vi "TEST - Remove Duplicates from 1D Array.vi"(8 "error in (no error)":errorcluster) -> (0 "error out":errorcluster, 2 "Pass?":bool=TRUE)   [LabVIEW 2020]
doc: "This VI template can be used for the functional testing of VIs; this implementation includes handling for the testing of polymorphic VIs, and the polymorphic elements should be removed if not needed.\n\nCoded by Douglas A. Femec, January 24, 2006.\n\nCopyright (c) 2005-2006 MKS Instruments, Inc.\nAll rights reserved."
uses:
  TEST - Remove Duplicates from 1D Array - Inputs.ctl
  Polymorphizer+ Data Type.ctl
  TEST - Remove Duplicates from 1D Array - Outputs.ctl
  source/library/Remove Duplicates from 1D Array/Remove Duplicates from 1D Array (EXT).vi
  source/library/Remove Duplicates from 1D Array/Remove Duplicates from 1D Array (I64).vi
  source/library/Remove Duplicates from 1D Array/Remove Duplicates from 1D Array (U64).vi
  source/library/Remove Duplicates from 1D Array/Remove Duplicates from 1D Array (LVObject).vi
  source/library/Remove Duplicates from 1D Array/Remove Duplicates from 1D Array (DBL).vi
  source/library/Remove Duplicates from 1D Array/Remove Duplicates from 1D Array (SGL).vi
  source/library/Remove Duplicates from 1D Array/Remove Duplicates from 1D Array (I32).vi
  source/library/Remove Duplicates from 1D Array/Remove Duplicates from 1D Array (I16).vi
  source/library/Remove Duplicates from 1D Array/Remove Duplicates from 1D Array (I8).vi
  source/library/Remove Duplicates from 1D Array/Remove Duplicates from 1D Array (U32).vi
  source/library/Remove Duplicates from 1D Array/Remove Duplicates from 1D Array (U16).vi
  source/library/Remove Duplicates from 1D Array/Remove Duplicates from 1D Array (U8).vi
  source/library/Remove Duplicates from 1D Array/Remove Duplicates from 1D Array (CXT).vi
  source/library/Remove Duplicates from 1D Array/Remove Duplicates from 1D Array (CDB).vi
  source/library/Remove Duplicates from 1D Array/Remove Duplicates from 1D Array (CSG).vi
  source/library/Remove Duplicates from 1D Array/Remove Duplicates from 1D Array (String).vi
  source/library/Remove Duplicates from 1D Array/Remove Duplicates from 1D Array (Path).vi
  source/library/Remove Duplicates from 1D Array/Remove Duplicates from 1D Array (Variant).vi
  source/library/Remove Duplicates from 1D Array/Remove Duplicates from 1D Array (Boolean).vi
  TestClass/TestClass.lvclass
panel:
  out "Generated Outputs":T1[][](array[typedef]) {"Duplicate-Free Array Out" format="%.2f"}
  in  "Expected Outputs":T1[](array[typedef])=[{"Description"="Expect empty array", "Duplicate-Free Array Out"=[], "Indices of Removed Elements"=[]}, {"Description"="Array with one element kept", "Duplicate-Free Array Out"=[1.0], "Indices of Removed Elements"=[]}, {"Description"="Expect one each of doubled elements kept", "Duplicate-Free Array Out"=[1.0, 0.0], "Indices of Removed Elements"=[2, 3]}, {"Description"="Expect array with one of each element", "Duplicate-Free Array Out"=[0.0, 1.0], "Indices of Removed Elements"=[]}, {"Description"="Expect array with one element", "Duplicate-Free Array Out"=[1.0], "Indices of Removed Elements"=[1, 2, 3]}] {"Duplicate-Free Array Out" format="%.2f"}
  in  "Inputs":T2[](array[typedef])=[{"Description"="Empty array", "Data Types to Test"=[enum."EXT", enum."DBL", enum."SGL", enum."I32", enum."I16", enum."I8", enum."U32", enum."U16", enum."U8", enum."CXT", enum."CDB", enum."CSG", enum."String", enum."Path", enum."Variant", enum."Boolean", enum."I64", enum."U64", enum."LabVIEW Object"], "Array In"=[]}, {"Description"="Array with one element", "Data Types to Test"=[enum."EXT", enum."DBL", enum."SGL", enum."I32", enum."I16", enum."I8", enum."U32", enum."U16", enum."U8", enum."CXT", enum."CDB", enum."CSG", enum."String", enum."Path", enum."Variant", enum."Boolean", enum."I64", enum."U64", enum."LabVIEW Object"], "Array In"=[1.0]}, {"Description"="Array with one each of doubled elements", "Data Types to Test"=[enum."EXT", enum."DBL", enum."SGL", enum."I32", enum."I16", enum."I8", enum."U32", enum."U16", enum."U8", enum."CXT", enum."CDB", enum."CSG", enum."String", enum."Path", enum."Variant", enum."Boolean", enum."I64", enum."U64", enum."LabVIEW Object"], "Array In"=[1.0, 0.0, 1.0, 0.0]}, {"Description"="Array with one of each element", "Data Types to Test"=[enum."EXT", enum."DBL", enum."SGL", enum."I32", enum."I16", enum."I8", enum."U32", enum."U16", enum."U8", enum."CXT", enum."CDB", enum."CSG", enum."String", enum."Path", enum."Variant", enum."Boolean", enum."I64", enum."U64", enum."LabVIEW Object"], "Array In"=[0.0, 1.0]}, {"Description"="Array with four of one element", "Data Types to Test"=[enum."EXT", enum."DBL", enum."SGL", enum."I32", enum."I16", enum."I8", enum."U32", enum."U16", enum."U8", enum."CXT", enum."CDB", enum."CSG", enum."String", enum."Path", enum."Variant", enum."Boolean", enum."I64", enum."U64", enum."LabVIEW Object"], "Array In"=[1.0, 1.0, 1.0, 1.0]}] {"Array In" format="%.2f"}
  # "Copyright (c) 2005-2006 MKS Instruments, Inc.\nAll rights reserved."
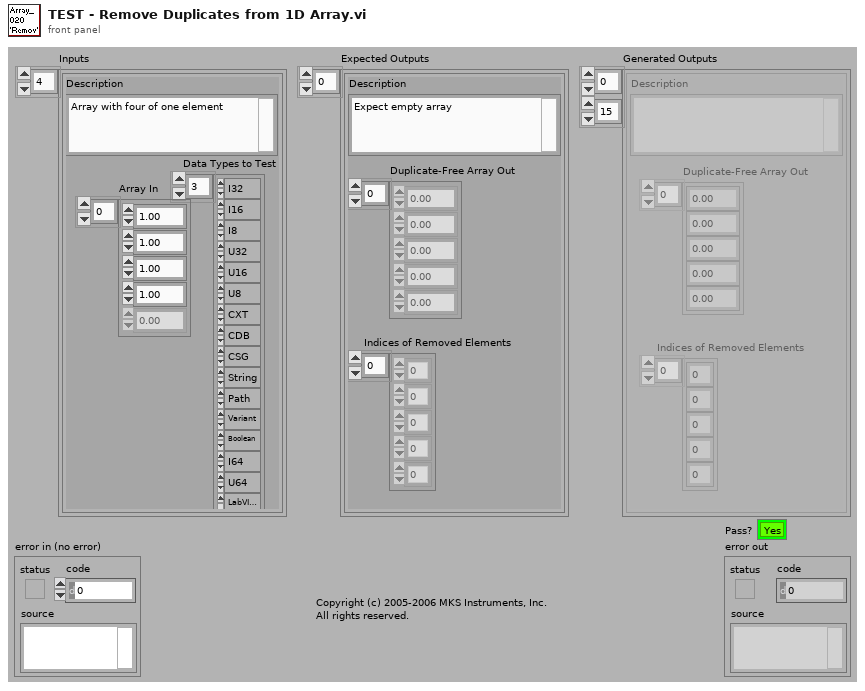
[diagram p1: front panel]
types:
  T1 = typedef "TEST - Remove Duplicates from 1D Array - Outputs.ctl" = cluster{"Description":string, "Duplicate-Free Array Out":sgl[], "Indices of Removed Elements":i32[]}
  T2 = typedef "TEST - Remove Duplicates from 1D Array - Inputs.ctl" = cluster{"Description":string, "Data Types to Test":T3[], "Array In":sgl[]}
  T3 = typedef "Polymorphizer+ Data Type.ctl" = enum16{"EXT", "DBL", "SGL", "I32", "I16", "I8", "U32", "U16", "U8", "CXT", "CDB", "CSG", "Boolean", "String", "Path", "Variant", "CTL-REF", "GEN-REF", "GObj-REF", "VI-REF", "ENUM", "ERR", "FILE-REF", "MENU-REF", "MENU-RING", "PICT-RING", "TXT&PICT-RING", "TXT-RING", "I64", "U64", "LabVIEW Object"}
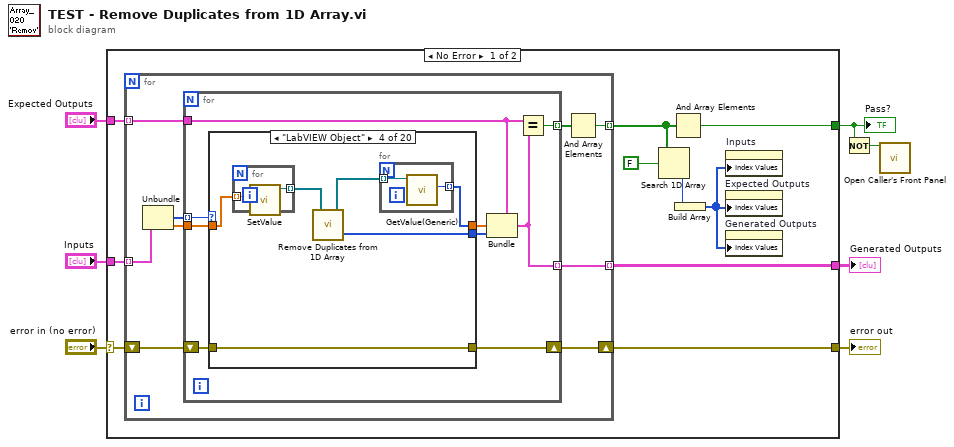
[diagram p0: block diagram]
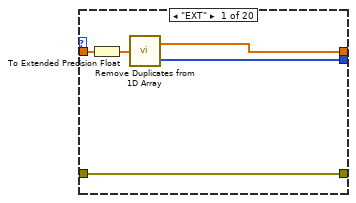
[diagram p2: hidden frame]
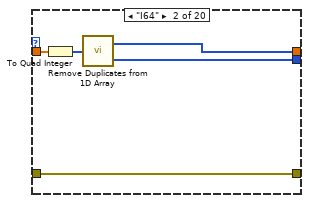
[diagram p3: hidden frame]
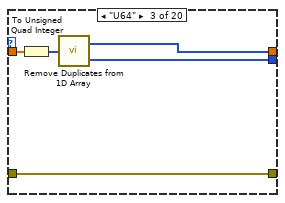
[diagram p4: hidden frame]
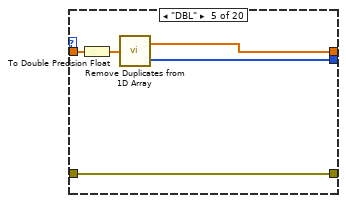
[diagram p5: hidden frame]
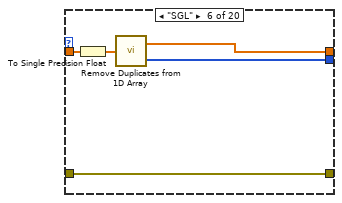
[diagram p6: hidden frame]
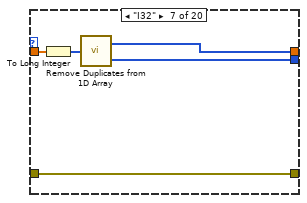
[diagram p7: hidden frame]
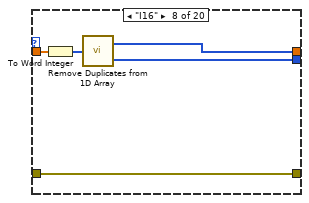
[diagram p8: hidden frame]
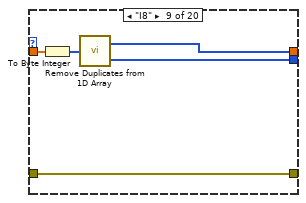
[diagram p9: hidden frame]
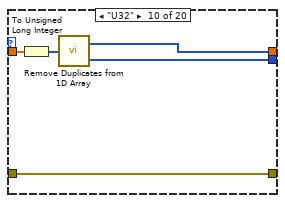
[diagram p10: hidden frame]
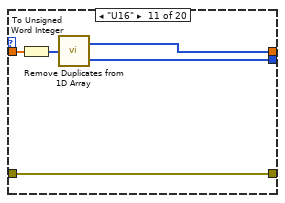
[diagram p11: hidden frame]
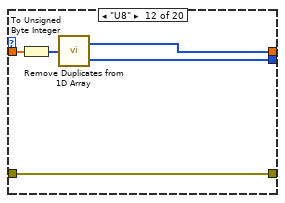
[diagram p12: hidden frame]
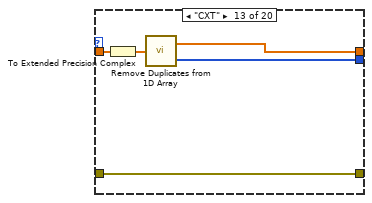
[diagram p13: hidden frame]
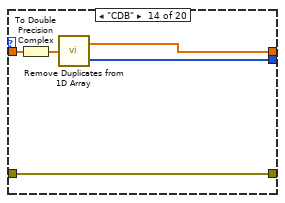
[diagram p14: hidden frame]
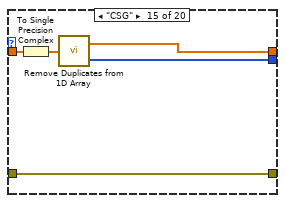
[diagram p15: hidden frame]
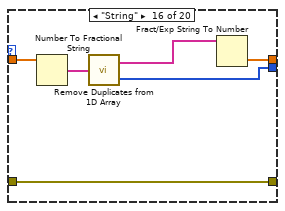
[diagram p16: hidden frame]
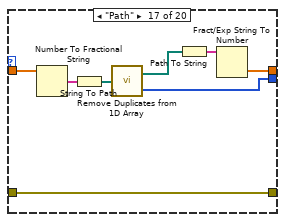
[diagram p17: hidden frame]
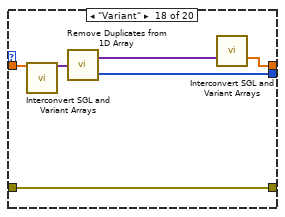
[diagram p18: hidden frame]
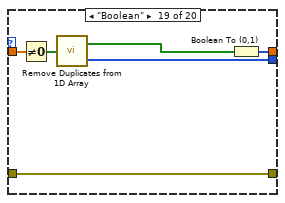
[diagram p19: hidden frame]
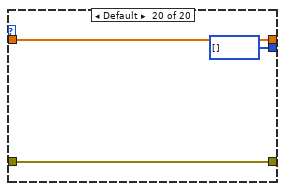
[diagram p20: hidden frame]
diagram:
  n1 = case shown="No Error" "error in (no error)" {
    selector: "error in (no error)" -> [w16 w145]
    tunnel: [w17 w145] -> w6
    tunnel: "Expected Outputs" -> [w14 _]
    tunnel: "Inputs" -> [w15 _]
    tunnel: [w13 _] -> w3
    tunnel: [w12 _] -> w2
    frame No Error {
      n2 = for {
        shift-right: [w21] -> w17
        shift-left: w16 -> [w22]
        tunnel: w15 -> [w23] mode=indexing
        tunnel: w14 -> [w26] mode=indexing
        tunnel: [w25] -> w13 mode=indexing
        tunnel: [w20] -> w11 mode=indexing
        n3 = Unbundle(w23) -> ("Data Types to Test"=w19:T3[], "Array In"=w18:sgl[])  [unwired: 1 out]
        n4 = for {
          tunnel: w26 -> [w35]
          tunnel: [w33] -> w25 mode=indexing
          tunnel: [w34] -> w24 mode=indexing
          shift-right: [w29] -> w21
          shift-left: w22 -> [w30]
          tunnel: w19 -> [w31] mode=indexing
          tunnel: w18 -> [w32]
          n5 = case shown="\"LabVIEW Object\"" w31 {
            tunnel: w32 -> [w37 w42 w47 w54 w62 w68 w73 w78 w82 w87 w92 w97 w103 w108 w113 w118 w124 w131 w137 w144]
            tunnel: [w39 w44 w49 w51 w64 w69 w74 w79 w84 w89 w94 w99 w104 w109 w114 w121 w128 w134 w140 w144] -> w27
            tunnel: w30 -> [w40 w45 w50 w56 w65 w70 w75 w80 w85 w90 w95 w100 w105 w110 w115 w120 w126 w135 w141 w143]
            tunnel: [w40 w45 w50 w56 w65 w70 w75 w80 w85 w90 w95 w100 w105 w110 w115 w120 w126 w135 w141 w143] -> w29
            tunnel: [w36 w41 w46 w55 w63 w66 w71 w76 w83 w88 w93 w98 w101 w106 w111 w116 w122 w130 w136 i32[] [] ("indices of removed elements")] -> w28
            frame "EXT" {
              n6 = To Extended Precision Float(1:w37) -> (0:w38:ext[])
              n7 = call-poly "Remove Duplicates from 1D Array.vi"("Input Array"=w38) -> ("Output Array"=w39:ext[], "indices of removed elements"=w36:i32[])
            }
            frame "I64" {
              n8 = To Quad Integer(1:w42) -> (0:w43:i64[])
              n9 = call-poly "Remove Duplicates from 1D Array.vi"("Input Array"=w43) -> ("Output Array"=w44:i64[], "indices of removed elements"=w41:i32[])
            }
            frame "U64" {
              n10 = To Unsigned Quad Integer(1:w47) -> (0:w48:u64[])
              n11 = call-poly "Remove Duplicates from 1D Array.vi"("Input Array"=w48) -> ("Output Array"=w49:u64[], "indices of removed elements"=w46:i32[])
            }
            frame "LabVIEW Object" {
              n12 = for {
                tunnel: w54 -> [w60] mode=indexing
                tunnel: [w59] -> w53 mode=indexing
                n13 = call "SetValue.vi"("Value"=w60) -> ("TestClass out"=w59:refnum<class "TestClass.lvclass">)  [unwired: 9 in, 1 out]
              }
              n14 = call-poly "Remove Duplicates from 1D Array.vi"("Input Array"=w53) -> ("Output Array"=w52:refnum<class>[], "indices of removed elements"=w55:i32[])
              n15 = for {
                tunnel: w52 -> [w58] mode=indexing
                tunnel: [w57] -> w51 mode=indexing
                n16 = call "GetValue(Generic).vi"("TestClass in"=w58) -> ("Value"=w57:i32)  [unwired: 8 in, 2 out]
              }
            }
            frame "DBL" {
              n17 = To Double Precision Float(number=w62) -> (double precision float=w61:dbl[])
              n18 = call-poly "Remove Duplicates from 1D Array.vi"("Input Array"=w61) -> ("Output Array"=w64:dbl[], "indices of removed elements"=w63:i32[])
            }
            frame "SGL" {
              n19 = To Single Precision Float(number=w68) -> (single precision float=w67:sgl[])
              n20 = call-poly "Remove Duplicates from 1D Array.vi"("Input Array"=w67) -> ("Output Array"=w69:sgl[], "indices of removed elements"=w66:i32[])
            }
            frame "I32" {
              n21 = To Long Integer(number=w73) -> (32bit integer=w72:i32[])
              n22 = call-poly "Remove Duplicates from 1D Array.vi"("Input Array"=w72) -> ("Output Array"=w74:i32[], "indices of removed elements"=w71:i32[])
            }
            frame "I16" {
              n23 = To Word Integer(number=w78) -> (16bit integer=w77:i16[])
              n24 = call-poly "Remove Duplicates from 1D Array.vi"("Input Array"=w77) -> ("Output Array"=w79:i16[], "indices of removed elements"=w76:i32[])
            }
            frame "I8" {
              n25 = To Byte Integer(number=w82) -> (8bit integer=w81:i8[])
              n26 = call-poly "Remove Duplicates from 1D Array.vi"("Input Array"=w81) -> ("Output Array"=w84:i8[], "indices of removed elements"=w83:i32[])
            }
            frame "U32" {
              n27 = To Unsigned Long Integer(number=w87) -> (unsigned 32bit integer=w86:u32[])
              n28 = call-poly "Remove Duplicates from 1D Array.vi"("Input Array"=w86) -> ("Output Array"=w89:u32[], "indices of removed elements"=w88:i32[])
            }
            frame "U16" {
              n29 = To Unsigned Word Integer(number=w92) -> (unsigned 16bit integer=w91:u16[])
              n30 = call-poly "Remove Duplicates from 1D Array.vi"("Input Array"=w91) -> ("Output Array"=w94:u16[], "indices of removed elements"=w93:i32[])
            }
            frame "U8" {
              n31 = To Unsigned Byte Integer(number=w97) -> (unsigned 8bit integer=w96:u8[])
              n32 = call-poly "Remove Duplicates from 1D Array.vi"("Input Array"=w96) -> ("Output Array"=w99:u8[], "indices of removed elements"=w98:i32[])
            }
            frame "CXT" {
              n33 = To Extended Precision Complex(1:w103) -> (0:w102:cxt[])
              n34 = call-poly "Remove Duplicates from 1D Array.vi"("Input Array"=w102) -> ("Output Array"=w104:cxt[], "indices of removed elements"=w101:i32[])
            }
            frame "CDB" {
              n35 = To Double Precision Complex(1:w108) -> (0:w107:cdb[])
              n36 = call-poly "Remove Duplicates from 1D Array.vi"("Input Array"=w107) -> ("Output Array"=w109:cdb[], "indices of removed elements"=w106:i32[])
            }
            frame "CSG" {
              n37 = To Single Precision Complex(1:w113) -> (0:w112:csg[])
              n38 = call-poly "Remove Duplicates from 1D Array.vi"("Input Array"=w112) -> ("Output Array"=w114:csg[], "indices of removed elements"=w111:i32[])
            }
            frame "String" {
              n39 = Number To Fractional String(number=w118) -> (F-format string=w117:string[])  [unwired: 3 in]
              n40 = call-poly "Remove Duplicates from 1D Array.vi"("Input Array"=w117) -> ("Output Array"=w119:string[], "indices of removed elements"=w116:i32[])
              n41 = Fract/Exp String To Number(string=w119) -> (number=w121:dbl[])  [unwired: 3 in, 1 out]
            }
            frame "Path" {
              n42 = Number To Fractional String(number=w124) -> (F-format string=w129:string[])  [unwired: 3 in]
              n43 = String To Path(string=w129) -> (path=w123:path[])
              n44 = call-poly "Remove Duplicates from 1D Array.vi"("Input Array"=w123) -> ("Output Array"=w125:path[], "indices of removed elements"=w122:i32[])
              n45 = Path To String(path=w125) -> (string=w127:string[])
              n46 = Fract/Exp String To Number(string=w127) -> (number=w128:dbl[])  [unwired: 3 in, 1 out]
            }
            frame "Variant" {
              n47 = call "Interconvert SGL and Variant Arrays.vi"("SGL 1D Array In"=w131) -> ("Variant 1D Array Out"=w132:variant[])  [unwired: 10 in, 4 out]
              n48 = call-poly "Remove Duplicates from 1D Array.vi"("Input Array"=w132) -> ("Output Array"=w133:variant[], "indices of removed elements"=w130:i32[])
              n49 = call "Interconvert SGL and Variant Arrays.vi"("Variant 1D Array In"=w133) -> ("SGL 1D Array Out"=w134:sgl[])  [unwired: 10 in, 4 out]
            }
            frame "Boolean" {
              n50 = Not Equal To 0?(x=w137) -> (x != 0?=w138:bool[])
              n51 = call-poly "Remove Duplicates from 1D Array.vi"("Input Array"=w138) -> ("Output Array"=w139:bool[], "indices of removed elements"=w136:i32[])
              n52 = Boolean To (0,1)(Boolean=w139) -> (0, 1=w140:i16[])
            }
            frame Default {
            }
          }
          n53 = Bundle(cluster=w35, "Duplicate-Free Array Out"=w27, "Indices of Removed Elements"=w28) -> (w33:T1)  [unwired: 1 in]
          n54 = Equal?(x=w35, y=w33) -> (x = y?=w34:bool)
        }
        n55 = And Array Elements(Boolean array=w24) -> (logical AND=w20:bool)
      }
      n56 = Search 1D Array(1D array=w11, element=FALSE) -> (index of element=w9:i32)  [unwired: 1 in]
      n57 = And Array Elements(Boolean array=w11) -> (logical AND=w12:bool)
      n58 = Build Array(w9) -> (w8:i32[])
      n59 = property on="Inputs" class="Arr (strict)"("Index Values"=w8) -> ()  [unwired: 2 in, 2 out]
      n60 = property on="Expected Outputs" class="Arr (strict)"("Index Values"=w8) -> ()  [unwired: 2 in, 2 out]
      n61 = property on="Generated Outputs" class="Arr (strict)"("Index Values"=w8) -> ()  [unwired: 2 in, 2 out]
    }
    frame Error {
    }
  }
  "error out" <- w6
  "Pass?" <- w2
  "Generated Outputs" <- w3
  n62 = Not(x=w2) -> (.not. x?=w1:bool)
  n63 = call "Open Caller's Front Panel.vi"("Open?"=w1) -> ()  [unwired: 14 in, 1 out]
